vi "TestDownlink Addon.vi"(0 "instrument handle":refnum<k15>, 1 "Channel DxSupply":string, 3 "FPGA Reference":refnum<k20>, 5 "error in (no error)":errorcluster, 6 "DL Tx Freq":i64, 7 "DL Tx  Power":dbl=-100.0, 9 "Resp Timeout (ms)":i32=500, 10 "DL Data Rate":dbl=600.0 format="%.2f", 11 "Active Dut":T1=enum."DUT 2") -> (13 "test_mode_resp":string, 14 "FPGA Ref Out":refnum<k20>, 15 "DL RSSI":i32, 17 "DL Rx Payload":string, 18 "Meas DL Idd":dbl, 19 "error out":errorcluster)   [LabVIEW 2018]
uses:
  Resources_Test/UART/ControlTestSlot.ctl
  <instrlib>/niRFSG/niRFSG.llb/niRFSG Ref Clock Sources.ctl
  SigFox 2015 - Monarch/RFSA e RFGA/SigFox Test.lvlib
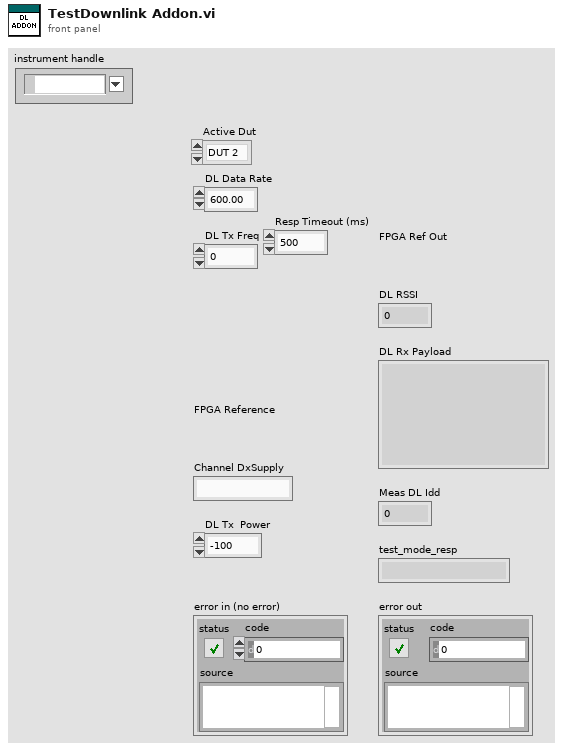
[diagram p1: front panel]
types:
  T1 = typedef "ControlTestSlot.ctl" = enum16{"DUT 1", "DUT 2"}
  T2 = typedef "niRFSG Ref Clock Sources.ctl" = string
  T3 = typedef "niAMT.lvlib/Complex Data Waveform.ctl" = cluster{"t0":dbl, "dt":dbl, "Y":cdb[]}
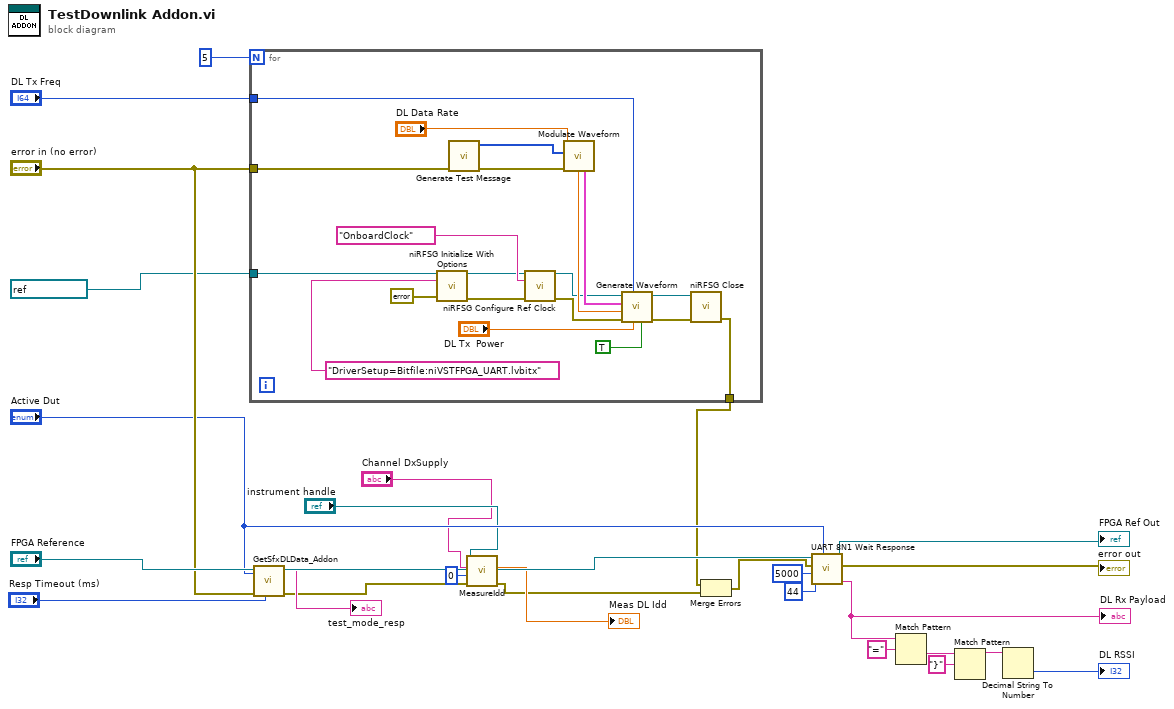
[diagram p0: block diagram]
diagram:
  n1 = for {
    N: 5 -> [_]
    tunnel: "error in (no error)" -> [w30]
    tunnel: [w29] -> w5
    tunnel: refnum<k15> "PXI1Slot5" ("RFSG Handle In") -> [w28]
    tunnel: "DL Tx Freq" -> [w27]
    n2 = call <instrlib>:"niRFSG Initialize With Options.vi"("resource name"=w28, "option string"="DriverSetup=Bitfile:niVSTFPGA_UART.lvbitx" ("Option String"), "error in"=errorcluster {"status"=FALSE, "code"=0, "source"=""}) -> ("instrument handle"=w44:refnum<k15>, "error out"=w43:errorcluster)  [unwired: 11 in]
    n3 = call "Generate Test Message.vi"("error in"=w30) -> ("error out"=w37:errorcluster, "Output Bit Stream"=w40:i8[])  [unwired: 9 in]
    n4 = call <instrlib>:"niRFSG Configure Ref Clock.vi"("instrument handle"=w44, "ref clock source"=T2 "OnboardClock" ("Clock Source"), "error in"=w43) -> ("instrument handle out"=w36:refnum<k15>, "error out"=w35:errorcluster)  [unwired: 11 in]
    n5 = call "Modulate Waveform.vi"("error in"=w37, "input bit stream"=w40, "Symbol Rate, Hz"="DL Data Rate") -> ("Signal Bandwidth"=w41:dbl, "output complex waveform"=w39:T3)  [unwired: 5 in, 2 out]
    n6 = call "Generate Waveform.vi"("Boolean"=TRUE, "Power Level (dBm)"="DL Tx  Power", "Center Frequency (Hz)"=w27, "error in (no error)"=w35, "Signal Bandwidth (Hz)"=w41, "IQ waveform"=w39, "IVI Refnum in"=w36) -> ("error out"=w33:errorcluster, "IVI Refnum out"=w32:refnum<k15>)  [unwired: 3 in]
    n7 = call <instrlib>:"niRFSG Close.vi"("instrument handle"=w32, "error in"=w33) -> ("error out"=w29:errorcluster)  [unwired: 13 in]
  }
  n8 = call "GetSfxDLData_Addon.vi"("Resp Timeout (ms)"="Resp Timeout (ms)", "Active Dut"="Active Dut", "Error In"="error in (no error)", "FPGA Reference"="FPGA Reference") -> ("Error Out"=w8:errorcluster, "test_mode_resp"=→"test_mode_resp":string)  [unwired: 5 in, 1 out]
  n9 = call "MeasureIdd.vi"("error in (no error)"=w8, "Deep Sleep Time"=u32 0, "channel name"="Channel DxSupply", "instrument handle"="instrument handle") -> ("error out"=w6:errorcluster, "Idd Average"=→"Meas DL Idd":dbl)  [unwired: 5 in, 1 out]
  n10 = Merge Errors(w5, w6) -> (w4:errorcluster)
  n11 = call "UART 8N1 Wait Response.vi"("Active Dut"="Active Dut", "Response Size (char)"=u32 44, "Response Timeout (ms)"=5000, "Error In"=w4, "FPGA VI Reference In"="FPGA Reference") -> ("Received Text"=w21:string, "Error Out"=→"error out":errorcluster, "FPGA VI Reference Out"=→"FPGA Ref Out":refnum<k20>)  [unwired: 2 in, 2 out]
  "DL Rx Payload" <- w21
  n12 = Match Pattern(string=w21, regular expression="=") -> (after substring=w12:string)  [unwired: 1 in, 3 out]
  n13 = Match Pattern(string=w12, regular expression="}") -> (before substring=w14:string)  [unwired: 1 in, 3 out]
  n14 = Decimal String To Number(string=w14) -> (number=→"DL RSSI":i32)  [unwired: 2 in, 1 out]
